vi "SubVI_Protocol_Testing.vi"(0 "TCP Network Connection in":refnum<k5>, 1 "Current level":dbl, 3 "Rest Period":i32=5000, 4 "Max Position":dbl, 5 "error in (no error)":errorcluster, 6 "Target Array":dbl[](array[numeric]), 7 "milliseconds to wait":u32, 9 "MidOut Proportion":dbl=0.6 format="%#_13g", 10 "Arm":string="right", 11 "Fixate Limit":dbl, 12 "Task":i32, 13 "MODE":string, 15 "Move Limit":dbl, 17 "ATAN Limit":dbl=2.0 format="%#_13g", 18 "Imagine Minimum Window":dbl) -> (14 "TCP Network Connection out":refnum<k5>, 19 "error out":errorcluster)   [LabVIEW 2020]
uses:
  Global 1.vi
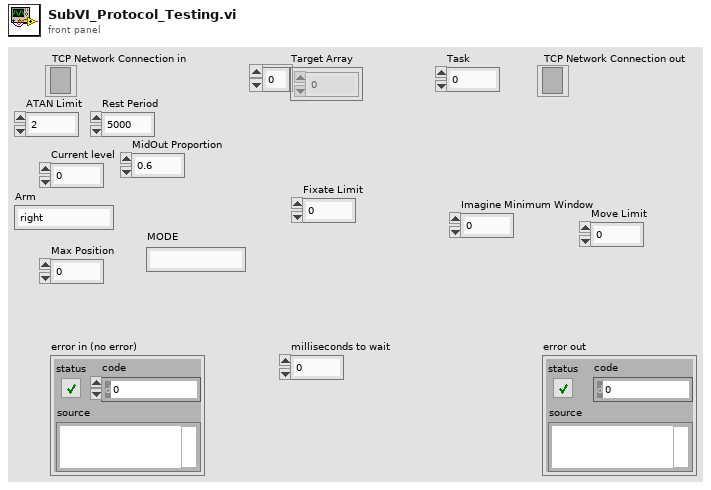
[diagram p1: front panel]
types:
  T1 = enum16{"Standard", "Buffered", "CRLF", "Immediate"}
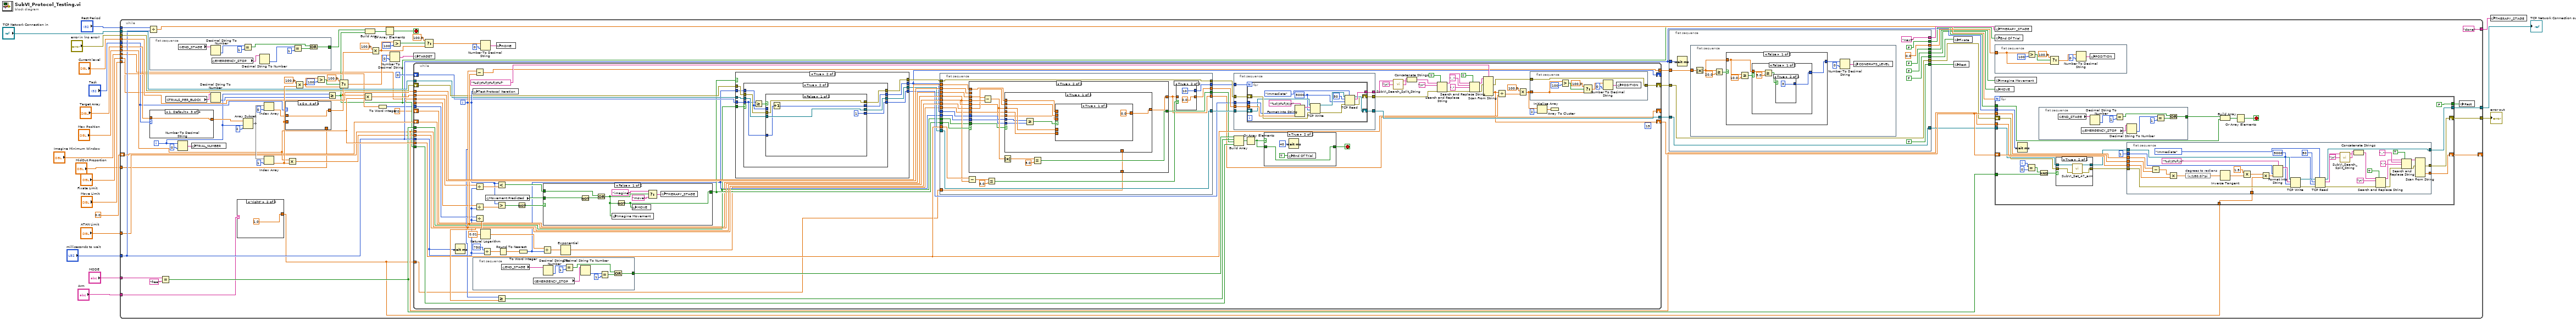
[diagram p0: block diagram]
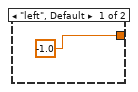
[diagram p2: hidden frame]
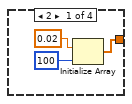
[diagram p3: hidden frame]
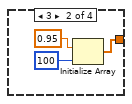
[diagram p4: hidden frame]
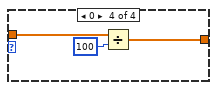
[diagram p5: hidden frame]
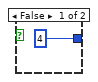
[diagram p6: hidden frame]
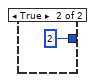
[diagram p7: hidden frame]
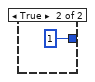
[diagram p8: hidden frame]
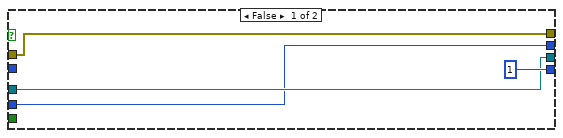
[diagram p10: hidden frame]
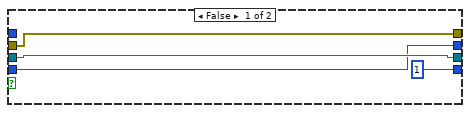
[diagram p11: hidden frame]
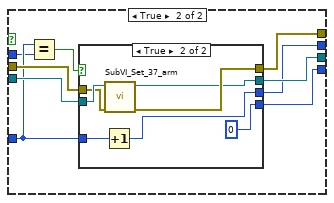
[diagram p12: hidden frame]
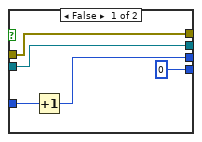
[diagram p13: hidden frame]
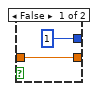
[diagram p15: hidden frame]
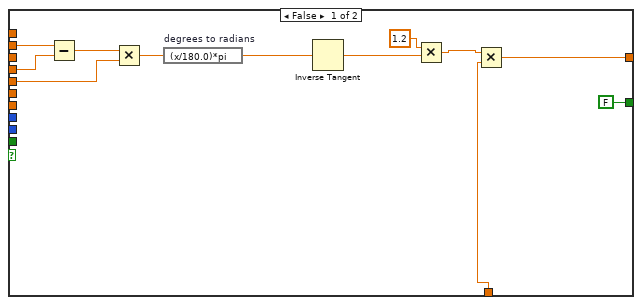
[diagram p16: hidden frame]
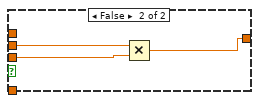
[diagram p17: hidden frame]
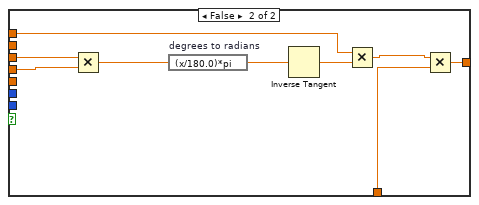
[diagram p18: hidden frame]
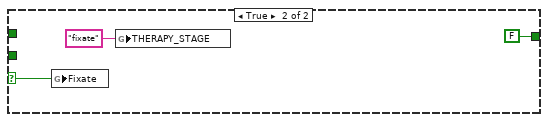
[diagram p19: hidden frame]
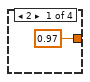
[diagram p20: hidden frame]
diagram:
  n1 = while {
    tunnel: "TCP Network Connection in" -> [w66]
    tunnel: "error in (no error)" -> [w67]
    tunnel: [w61] -> w9
    tunnel: "milliseconds to wait" -> [w53]
    tunnel: "Task" -> [w36]
    tunnel: "Target Array" -> [w38]
    tunnel: ["done" ("THERAPY_STAGE")] -> w10
    tunnel: [w62] -> w11
    tunnel: "Max Position" -> [w64]
    tunnel: "Current level" -> [w63]
    shift-right: [w59] -> _
    shift-left: 0.0 -> [w60]
    tunnel: "ATAN Limit" -> [w30]
    tunnel: "Move Limit" -> [w44]
    tunnel: "Imagine Minimum Window" -> [w27]
    tunnel: "Fixate Limit" -> [w25]
    tunnel: "MODE" -> [w42]
    tunnel: "Rest Period" -> [w28]
    tunnel: "Arm" -> [w22]
    tunnel: "MidOut Proportion" -> [w21]
    i -> [w33]
    stop <- w31 stop-if-true
    n2 = Divide(x=w28, y=w53) -> (x/y=w52:dbl)
    n3 = flat-sequence {
      tunnel: [w471] -> w34
      frame #0 {
        n4 = global read "Global 1.vi" "END_STAGE"() -> (w479:string)
        n5 = Decimal String To Number(string=w479) -> (number=w478:i32)  [unwired: 2 in, 1 out]
        n6 = global read "Global 1.vi" "EMERGENCY_STOP"() -> (w474:string)
        n7 = Equal?(x=w478, y=1) -> (x = y?=w472:bool)
        n8 = Decimal String To Number(string=w474) -> (number=w476:i32)  [unwired: 2 in, 1 out]
        n9 = Equal?(x=w476, y=1) -> (x = y?=w473:bool)
        n10 = Or(x=w472, y=w473) -> (x .or. y?=w471:bool)
      }
    }
    n11 = case shown="1, Default" w36 {
      tunnel: w38 -> [_ _ w104 w107]
      tunnel: [w98 w101 w104 w105] -> w37
      frame 2 {
        n12 = Initialize Array(0.02 ("element"), 100 ("dimension size")) -> (w98:dbl[])
      }
      frame 3 {
        n13 = Initialize Array(0.95 ("element"), 100 ("dimension size")) -> (w101:dbl[])
      }
      frame 1, Default {
      }
      frame 0 {
        n14 = Divide(x=w107, y=100) -> (x/y=w105:dbl[])
      }
    }
    n15 = Equal?(x=w42, y="free") -> (x = y?=w40:bool)
    n16 = global read "Global 1.vi" "TRIALS_PER_BLOCK"() -> (w32:string)
    n17 = Number To Decimal String(number=w33, width (-)=i16 0) -> (decimal integer string=w70:string)
    n18 = global write "Global 1.vi" "TRIAL_NUMBER"(w70) -> ()
    n19 = Decimal String To Number(string=w32) -> (number=w26:i32)  [unwired: 2 in, 1 out]
    n20 = case shown="\"right\"" w22 {
      tunnel: [-1.0 1.0] -> w23
      frame "left", Default {
      }
      frame "right" {
      }
    }
    n21 = Array Subset(array=w37, index=w33, length=2) -> (w94:dbl[])
    n22 = Index Array(array=w94, index=0) -> (element=w73:dbl)
    n23 = Index Array(array=w94, index=1) -> (element=w74:dbl)
    n24 = case shown="0" w36 {
      tunnel: [0.97 0.02 w489 w490] -> w72
      tunnel: w74 -> [_ _ _ _]
      tunnel: w73 -> [_ _ _ w490]
      tunnel: w21 -> [_ _ w489 _]
      frame 2 {
      }
      frame 3 {
      }
      frame 1, Default {
      }
      frame 0 {
      }
    }
    n25 = Multiply(x=w64, y=w74) -> (x*y=w39:dbl)
    n26 = Multiply(x=100.0, y=w74) -> (x*y=w86:dbl)
    n27 = Greater?(x=w86, y=100) -> (0:w90:bool)
    n28 = Greater Or Equal?(x=w33, y=w26) -> (x >= y?=w29:bool)
    n29 = Select(t=100.0, s=w90, f=w86) -> (s? t:f=w91:dbl)
    n30 = Multiply(x=w72, y=w64) -> (x*y=w65:dbl)
    n31 = Build Array(w34, w29) -> (w35:bool[])
    n32 = Multiply(x=100.0, y=w72) -> (x*y=w79:dbl)
    n33 = To Word Integer(number=w44) -> (16bit integer=w20:i16)
    n34 = Or Array Elements(Boolean array=w35) -> (logical OR=w31:bool)
    n35 = Number To Decimal String(number=w91, width (-)=i16 0) -> (decimal integer string=w76:string)
    n36 = Greater?(x=w79, y=100) -> (0:w83:bool)
    n37 = global write "Global 1.vi" "TARGET"(w76) -> ()
    n38 = while {
      tunnel: [w265] -> w54
      shift-right: [w230] -> w56
      shift-left: w67 -> [w243]
      tunnel: w66 -> [w241]
      tunnel: w53 -> [w221]
      tunnel: w65 -> [w258]
      tunnel: w39 -> [w255]
      tunnel: w64 -> [w264]
      shift-right: [w259] -> w58
      shift-left: w60 -> [w254]
      tunnel: w63 -> [w263]
      tunnel: w30 -> [w256]
      tunnel: [w253] -> w46
      tunnel: w20 -> [w247]
      tunnel: w27 -> [w246]
      tunnel: w25 -> [w245]
      tunnel: w40 -> [w228]
      shift-right: [w227] -> _
      shift-left: 0 -> [w238]
      tunnel: w29 -> [w235]
      shift-right: [w226] -> _
      shift-left: 0.0 -> [w225]
      tunnel: w23 -> [w215]
      i -> [w244]
      stop <- w236 stop-if-true
      (unwired) 15 ("y")
      n39 = Wait (ms)(milliseconds to wait=w221) -> ()  [unwired: 1 out]
      n40 = global write "Global 1.vi" "Test Protocol Iteration"(w244) -> ()
      n41 = flat-sequence {
        tunnel: [w443] -> w252
        frame #0 {
          n42 = global read "Global 1.vi" "END_STAGE"() -> (w451:string)
          n43 = global read "Global 1.vi" "EMERGENCY_STOP"() -> (w446:string)
          n44 = Decimal String To Number(string=w451) -> (number=w450:i32)  [unwired: 2 in, 1 out]
          n45 = Equal?(x=w450, y=1) -> (x = y?=w444:bool)
          n46 = Decimal String To Number(string=w446) -> (number=w448:i32)  [unwired: 2 in, 1 out]
          n47 = Equal?(x=w448, y=1) -> (x = y?=w445:bool)
          n48 = Or(x=w444, y=w445) -> (x .or. y?=w443:bool)
        }
      }
      n49 = Subtract(x=w255, y=w254) -> (x-y=w253:dbl)
      n50 = Divide(x=w246, y=w221) -> (x/y=w287:dbl)
      n51 = Divide(x=w245, y=w221) -> (x/y=w288:dbl)
      n52 = Divide(x=w247, y=w221) -> (x/y=w289:dbl)
      n53 = Natural Logarithm(1:0.01 ("y")) -> (0:w223:dbl)
      n54 = Divide(x=750, y=w221) -> (x/y=w218:dbl)
      n55 = global read "Global 1.vi" "Movement Predicted"() -> (w257:bool)
      n56 = Less?(x=w244, y=w287) -> (x < y?=w267:bool)
      n57 = Greater?(x=w244, y=w288) -> (0:w286:bool)
      n58 = Greater Or Equal?(x=w244, y=w289) -> (x >= y?=w251:bool)
      n59 = Round To Nearest(number=w218) -> (nearest integer value=w219:dbl)
      n60 = Not(x=w286) -> (.not. x?=w268:bool)
      n61 = To Word Integer(number=w219) -> (16bit integer=w217:i16)
      n62 = Divide(x=w223, y=w217) -> (x/y=w222:dbl)
      n63 = case shown="False" w268 {
        selector: w268 -> [_ w468]
        tunnel: w257 -> [w466 _]
        tunnel: w267 -> [w465 _]
        tunnel: [w461 FALSE] -> w237
        frame False {
          n64 = Not(x=w466) -> (.not. x?=w460:bool)
          n65 = Or(x=w465, y=w460) -> (x .or. y?=w462:bool)
          n66 = global write "Global 1.vi" "Imagine Movement"(w462) -> ()
          n67 = Not(x=w462) -> (.not. x?=w461:bool)
          n68 = global write "Global 1.vi" "MOVE"(w461) -> ()
          n69 = Select(t="imagine" ("THERAPY_STAGE"), s=w462, f="move" ("THERAPY_STAGE")) -> (s? t:f=w467:string)
          n70 = global write "Global 1.vi" "THERAPY_STAGE"(w467) -> ()
        }
        frame True {
          n71 = global write "Global 1.vi" "Fixate"(w468) -> ()
          n72 = global write "Global 1.vi" "THERAPY_STAGE"("fixate" ("THERAPY_STAGE")) -> ()
        }
      }
      n73 = Exponential(1:w222) -> (0:w216:dbl)
      n74 = case shown="True" w237 {
        tunnel: w243 -> [w292 w302]
        tunnel: [1 ("input 1") w299] -> w242
        tunnel: w241 -> [w291 w296]
        tunnel: [w291 w297] -> w240
        tunnel: [w292 w301] -> w239
        tunnel: w238 -> [w290 w295]
        tunnel: [w290 w300] -> w227
        tunnel: w228 -> [_ w298]
        tunnel: w217 -> [_ w294]
        frame False {
        }
        frame True {
          n75 = case shown="True" w298 {
            tunnel: w302 -> [w306 w315]
            tunnel: w296 -> [w305 w314]
            tunnel: [w305 w313] -> w297
            tunnel: [w306 w312] -> w301
            tunnel: [w303 w311] -> w300
            tunnel: [1 ("input 1") w310] -> w299
            tunnel: w295 -> [w303 w308]
            tunnel: w294 -> [_ w307]
            frame False {
            }
            frame True {
              n76 = Greater Or Equal?(x=w308, y=w307) -> (x >= y?=w309:bool)
              n77 = case shown="False" w309 {
                tunnel: w314 -> [w319 w329]
                tunnel: w315 -> [w320 w328]
                tunnel: [w320 w327] -> w312
                tunnel: [w319 w326] -> w313
                tunnel: [w316 w325] -> w311
                tunnel: [1 ("input 1") w324] -> w310
                tunnel: w308 -> [w317 w323]
                tunnel: w307 -> [_ w322]
                frame False {
                  n78 = Increment(x=w317) -> (x+1=w316:i32)
                }
                frame True {
                  n79 = Equal?(x=w323, y=w322) -> (x = y?=w321:bool)
                  n80 = case shown="True" w321 {
                    tunnel: w329 -> [w332 w341]
                    tunnel: w328 -> [w331 w340]
                    tunnel: [w331 w339] -> w327
                    tunnel: [w332 w338] -> w326
                    tunnel: [w334 w337] -> w325
                    tunnel: [0 ("input 1") 0 ("input 1")] -> w324
                    tunnel: w323 -> [w333 w335]
                    frame False {
                      n81 = Increment(x=w333) -> (x+1=w334:i32)
                    }
                    frame True {
                      n82 = Increment(x=w335) -> (x+1=w337:i32)
                      n83 = call "SubVI_Set_37_arm.vi"("error in (no error)"=w340, "TCP Network Connection in"=w341) -> ("error out"=w339:errorcluster, "TCP Network Connection out"=w338:refnum<k5>)  [unwired: 8 in]
                    }
                  }
                }
              }
            }
          }
        }
      }
      n84 = flat-sequence {
        tunnel: w239 -> [w367]
        tunnel: w240 -> [w366]
        tunnel: w258 -> [w365]
        tunnel: w255 -> [w364]
        tunnel: [w363] -> w261
        tunnel: [w367] -> w260
        tunnel: [w366] -> w262
        tunnel: w254 -> [w354]
        tunnel: w264 -> [w360]
        tunnel: w263 -> [w359]
        tunnel: w237 -> [w358]
        tunnel: w256 -> [w357]
        tunnel: [w356] -> w250
        tunnel: [w355] -> w229
        tunnel: w228 -> [w352]
        tunnel: w227 -> [w351]
        tunnel: w217 -> [w350]
        tunnel: [w349] -> w226
        tunnel: w225 -> [w348]
        tunnel: w216 -> [w347]
        tunnel: w215 -> [w346]
        frame #0 {
          n85 = Subtract(x=w360, y=w354) -> (x-y=w362:dbl)
          n86 = case shown="True" w358 {
            tunnel: w365 -> [w377 _]
            tunnel: w364 -> [_ w395]
            tunnel: w354 -> [w382 w398]
            tunnel: w359 -> [_ w396]
            tunnel: [w378 w397] -> w349
            tunnel: w357 -> [w374 w391]
            tunnel: [FALSE w390] -> w356
            tunnel: w352 -> [_ w389]
            tunnel: w351 -> [_ w388]
            tunnel: w350 -> [_ w387]
            tunnel: w348 -> [_ w386]
            tunnel: w347 -> [_ w385]
            tunnel: w346 -> [w372 w384]
            frame False {
              n87 = Subtract(x=w377, y=w382) -> (x-y=w376:dbl)
              n88 = Multiply(x=w376, y=w374) -> (x*y=w375:dbl)
              n89 = expression code="(x/180.0)*pi" "degrees to radians"(w375) -> (w383:dbl)
              n90 = Inverse Tangent(1:w383) -> (0:w381:dbl)
              n91 = Multiply(x=1.2, y=w381) -> (x*y=w379:dbl)
              n92 = Multiply(x=w379, y=w372) -> (x*y=w378:dbl)
            }
            frame True {
              n93 = Subtract(x=w395, y=w398) -> (x-y=w392:dbl)
              n94 = Absolute Value(x=w392) -> (abs(x)=w394:dbl)
              n95 = case shown="True" w389 {
                tunnel: [w407 w417] -> w397
                tunnel: w396 -> [w406 w416]
                tunnel: w392 -> [w405 w415]
                tunnel: w391 -> [w404 w413]
                tunnel: w388 -> [w403 _]
                tunnel: w387 -> [w402 _]
                tunnel: w386 -> [w400 _]
                tunnel: w385 -> [w399 _]
                tunnel: w384 -> [_ w412]
                frame True {
                  n96 = Greater Or Equal?(x=w403, y=w402) -> (x >= y?=w401:bool)
                  n97 = case shown="True" w401 {
                    tunnel: [0.0 w411] -> w407
                    tunnel: w406 -> [_ _]
                    tunnel: w405 -> [_ _]
                    tunnel: w404 -> [_ _]
                    tunnel: w400 -> [_ w410]
                    tunnel: w399 -> [_ w409]
                    frame True {
                    }
                    frame False {
                      n98 = Multiply(x=w410, y=w409) -> (x*y=w411:dbl)
                    }
                  }
                }
                frame False {
                  n99 = Multiply(x=w415, y=w413) -> (x*y=w414:dbl)
                  n100 = expression code="(x/180.0)*pi" "degrees to radians"(w414) -> (w420:dbl)
                  n101 = Inverse Tangent(1:w420) -> (0:w419:dbl)
                  n102 = Multiply(x=w416, y=w419) -> (x*y=w418:dbl)
                  n103 = Multiply(x=w418, y=w412) -> (x*y=w417:dbl)
                }
              }
              n104 = Less Or Equal?(x=w394, y=5.0) -> (x <= y?=w390:bool)
            }
          }
          n105 = Less Or Equal?(x=w362, y=3.0) -> (x <= y?=w353:bool)
          n106 = case shown="True" w353 {
            tunnel: w349 -> [w369 _]
            tunnel: [w369 0.0] -> w363
            tunnel: [1 10] -> w355
            frame False {
            }
            frame True {
            }
          }
        }
      }
      n107 = flat-sequence {
        tunnel: w261 -> [w428]
        tunnel: [w427] -> w266
        tunnel: [w426] -> w265
        tunnel: [w425] -> w234
        tunnel: w260 -> [w424]
        tunnel: w242 -> [w423]
        tunnel: w262 -> [w422]
        tunnel: w229 -> [w421]
        frame #0 {
          n108 = for {
            N: w421 -> [_]
            tunnel: w428 -> [w436]
            tunnel: [w435] -> w427
            tunnel: w423 -> [w431]
            shift-right: [w433] -> w425
            shift-left: w424 -> [w432]
            shift-right: [w434] -> w426
            shift-left: w422 -> [w430]
            w429 = 5000 ("timeout ms (25000)")
            n109 = Format Into String(format string="%d\\t%f\\t\\n", w431, w436) -> (resulting string=w437:string)  [unwired: 2 in, 1 out]
            n110 = TCP Write(connection ID=w430, data in=w437, error in (no error)=w432, 9:w429) -> (connection ID out=w440:refnum<k5>, error out=w439:errorcluster)  [unwired: 1 out]
            n111 = TCP Read(connection ID=w440, bytes to read=50, error in (no error)=w439, 7:T1."Immediate" ("mode (standard)"), 9:w429) -> (connection ID out=w434:refnum<k5>, data out=w435:string, error out=w433:errorcluster)
          }
        }
      }
      n112 = Build Array(w252, w251, w250, w235) -> (w249:bool[])
      n113 = Or Array Elements(Boolean array=w249) -> (logical OR=w248:bool)
      n114 = case shown="True" w248 {
        tunnel: w248 -> [w342 w345]
        tunnel: [w342 w345] -> w236
        frame False {
        }
        frame True {
          n115 = global write "Global 1.vi" "End Of Trial"(TRUE ("End Of Trial")) -> ()
          n116 = Wait (ms)(milliseconds to wait=u32 40) -> ()  [unwired: 1 out]
        }
      }
      n117 = call <userlib>:"SubVI_Search_Split_String.vi"("search string/char (-)"="\n", "string"=w266) -> ("substring after match"=w280:string, "substring before match"=w271:string)  [unwired: 1 in, 1 out]
      n118 = Concatenate Strings(w280, w271) -> (w277:string)
      n119 = Search and Replace String(replace all?=TRUE ("replace all? (F)"), input string=w277, search string="\n", error in=w234) -> (result string=w272:string, error out=w233:errorcluster)  [unwired: 4 in, 2 out]
      n120 = Search and Replace String(replace all?=TRUE ("replace all? (F)"), input string=w272, search string="..", replace string="." ("replace string (\"\")"), error in=w233) -> (result string=w270:string, error out=w232:errorcluster)  [unwired: 3 in, 2 out]
      n121 = Scan From String(format string="%d\\t%f\\t%f\\t%f", input string=w270, error in=w232) -> (error out=w231:errorcluster, output 3=w259:dbl)  [unwired: 8 in, 2 out]
      n122 = Divide(x=w259, y=w264) -> (x/y=w283:dbl)
      n123 = Multiply(x=100.0, y=w283) -> (x*y=w269:dbl)
      n124 = flat-sequence {
        tunnel: w269 -> [w453]
        tunnel: w231 -> [w452]
        tunnel: [w452] -> w230
        frame #0 {
          n125 = Greater?(x=w453, y=100) -> (0:w458:bool)
          n126 = Select(t=100.0, s=w458, f=w453) -> (s? t:f=w455:dbl)
          n127 = Number To Decimal String(number=w455, width (-)=i16 0) -> (decimal integer string=w454:string)
          n128 = global write "Global 1.vi" "POSITION"(w454) -> ()
        }
      }
      n129 = Initialize Array(w269, 2 ("dimension size")) -> (w284:dbl[])
      n130 = Array To Cluster(array=w284) -> ()  [unwired: 1 out]
    }
    n131 = Select(t=100.0, s=w83, f=w79) -> (s? t:f=w84:dbl)
    n132 = Number To Decimal String(number=w84, width (-)=i16 0) -> (decimal integer string=w77:string)
    n133 = global write "Global 1.vi" "HOME"(w77) -> ()
    n134 = flat-sequence {
      tunnel: [FALSE ("MOVE")] -> w49
      tunnel: [FALSE ("Imagine Movement")] -> w50
      tunnel: [TRUE ("Rest")] -> w47
      tunnel: [FALSE ("Fixate")] -> w51
      tunnel: ["next" ("THERAPY_STAGE")] -> w69
      tunnel: [0.0 ("Arm_position")] -> w68
      tunnel: w53 -> [w112]
      tunnel: [w111] -> w57
      tunnel: w56 -> [w111]
      tunnel: [w110] -> w55
      tunnel: w54 -> [w110]
      tunnel: w46 -> [w109]
      tunnel: [FALSE ("End Of Trial")] -> w45
      frame #0 {
        n135 = Wait (ms)(milliseconds to wait=w112) -> ()  [unwired: 1 out]
        n136 = flat-sequence {
          tunnel: w109 -> [w120]
          frame #0 {
            n137 = Absolute Value(x=w120) -> (abs(x)=w119:dbl)
            n138 = Greater Or Equal?(x=w119, y=20.0) -> (x >= y?=w124:bool)
            n139 = case shown="False" w124 {
              tunnel: [w127 1] -> w122
              tunnel: w119 -> [w126 _]
              frame False {
                n140 = Greater Or Equal?(x=w126, y=10.0) -> (x >= y?=w129:bool)
                n141 = case shown="False" w129 {
                  tunnel: [w131 2] -> w127
                  tunnel: w126 -> [w133 _]
                  frame False {
                    n142 = Greater Or Equal?(x=w133, y=5.0) -> (x >= y?=w130:bool)
                    n143 = case shown="True" w130 {
                      tunnel: [4 3] -> w131
                      frame False {
                      }
                      frame True {
                      }
                    }
                  }
                  frame True {
                  }
                }
              }
              frame True {
              }
            }
            n144 = Number To Decimal String(number=w122, width (-)=i16 0) -> (decimal integer string=w121:string)
            n145 = global write "Global 1.vi" "CONGRATS_LEVEL"(w121) -> ()
          }
        }
      }
    }
    n146 = global write "Global 1.vi" "Fixate"(w51) -> ()
    n147 = global write "Global 1.vi" "Rest"(w47) -> ()
    n148 = global write "Global 1.vi" "THERAPY_STAGE"(w69) -> ()
    n149 = global write "Global 1.vi" "End Of Trial"(w45) -> ()
    n150 = flat-sequence {
      tunnel: w68 -> [w480]
      frame #0 {
        n151 = Greater?(x=w480, y=100) -> (0:w485:bool)
        n152 = Select(t=100.0, s=w485, f=w480) -> (s? t:f=w482:dbl)
        n153 = Number To Decimal String(number=w482, width (-)=i16 0) -> (decimal integer string=w481:string)
        n154 = global write "Global 1.vi" "POSITION"(w481) -> ()
      }
    }
    n155 = global write "Global 1.vi" "Imagine Movement"(w50) -> ()
    n156 = global write "Global 1.vi" "MOVE"(w49) -> ()
    n157 = for {
      N: w52 -> [_]
      shift-right: [w158] -> w61
      shift-left: w57 -> [w146]
      tunnel: [FALSE ("Rest")] -> w48
      tunnel: w55 -> [w145]
      tunnel: [w157] -> w62
      shift-right: [w156] -> w59
      shift-left: w58 -> [w154]
      tunnel: w58 -> [w155]
      tunnel: w53 -> [w153]
      tunnel: w30 -> [w152]
      tunnel: w40 -> [w148]
      tunnel: w29 -> [w140]
      tunnel: w23 -> [w138]
      i -> [w151]
      stop <- w139 stop-if-true
      n158 = Wait (ms)(milliseconds to wait=w153) -> ()  [unwired: 1 out]
      n159 = Equal?(x=w151, y=0) -> (x = y?=w149:bool)
      n160 = flat-sequence {
        tunnel: [w167] -> w141
        frame #0 {
          n161 = global read "Global 1.vi" "END_STAGE"() -> (w175:string)
          n162 = global read "Global 1.vi" "EMERGENCY_STOP"() -> (w170:string)
          n163 = Decimal String To Number(string=w175) -> (number=w174:i32)  [unwired: 2 in, 1 out]
          n164 = Equal?(x=w174, y=1) -> (x = y?=w168:bool)
          n165 = Decimal String To Number(string=w170) -> (number=w172:i32)  [unwired: 2 in, 1 out]
          n166 = Equal?(x=w172, y=1) -> (x = y?=w169:bool)
          n167 = Or(x=w168, y=w169) -> (x .or. y?=w167:bool)
        }
      }
      n168 = And(x=w149, y=w148) -> (x .and. y?=w147:bool)
      n169 = case shown="True" w147 {
        tunnel: w145 -> [w161 w166]
        tunnel: w146 -> [w162 w165]
        tunnel: [w162 w164] -> w143
        tunnel: [w161 w163] -> w144
        frame False {
        }
        frame True {
          n170 = call "SubVI_Set_47_arm.vi"("error in (no error)"=w165, "TCP Network Connection in"=w166) -> ("error out"=w164:errorcluster, "TCP Network Connection out"=w163:refnum<k5>)  [unwired: 8 in]
        }
      }
      n171 = flat-sequence {
        tunnel: 1 ("input 1") -> [w208]
        tunnel: [w207] -> w157
        tunnel: [w178] -> w158
        tunnel: w144 -> [w206]
        tunnel: [w195] -> w156
        tunnel: w155 -> [w192]
        tunnel: w154 -> [w191]
        tunnel: w152 -> [w184]
        tunnel: w143 -> [w182]
        tunnel: w138 -> [w176]
        frame #0 {
          w177 = 5000 ("timeout ms (25000)")
          n172 = Subtract(x=w192, y=w191) -> (x-y=w185:dbl)
          n173 = Multiply(x=w185, y=w184) -> (x*y=w183:dbl)
          n174 = expression code="(x/180.0)*pi" "degrees to radians"(w183) -> (w187:dbl)
          n175 = Inverse Tangent(1:w187) -> (0:w186:dbl)
          n176 = Multiply(x=1.5, y=w186) -> (x*y=w189:dbl)
          n177 = Multiply(x=w189, y=w176) -> (x*y=w190:dbl)
          n178 = Format Into String(format string="%d\\t%f\\n", w208, w190) -> (resulting string=w209:string)  [unwired: 2 in, 1 out]
          n179 = TCP Write(connection ID=w206, data in=w209, error in (no error)=w182, 9:w177) -> (connection ID out=w212:refnum<k5>, error out=w211:errorcluster)  [unwired: 1 out]
          n180 = TCP Read(connection ID=w212, bytes to read=50, error in (no error)=w211, 7:T1."Immediate" ("mode (standard)"), 9:w177) -> (connection ID out=w207:refnum<k5>, data out=w196:string, error out=w181:errorcluster)
          n181 = call <userlib>:"SubVI_Search_Split_String.vi"("search string/char (-)"="\n", "string"=w196) -> ("substring after match"=w204:string, "substring before match"=w198:string)  [unwired: 1 in, 1 out]
          n182 = Concatenate Strings(w204, w198) -> (w202:string)
          n183 = Search and Replace String(replace all?=TRUE ("replace all? (F)"), input string=w202, search string="\n", error in=w181) -> (result string=w199:string, error out=w180:errorcluster)  [unwired: 4 in, 2 out]
          n184 = Search and Replace String(replace all?=TRUE ("replace all? (F)"), input string=w199, search string="..", replace string="." ("replace string (\"\")"), error in=w180) -> (result string=w197:string, error out=w179:errorcluster)  [unwired: 3 in, 2 out]
          n185 = Scan From String(input string=w197, error in=w179) -> (error out=w178:errorcluster, output 3=w195:dbl)  [unwired: 9 in, 2 out]
        }
      }
      n186 = Build Array(w141, w140) -> (w142:bool[])
      n187 = Or Array Elements(Boolean array=w142) -> (logical OR=w139:bool)
    }
    n188 = global write "Global 1.vi" "Rest"(w48) -> ()
  }
  "TCP Network Connection out" <- w11
  "error out" <- w9
  n189 = global write "Global 1.vi" "THERAPY_STAGE"(w10) -> ()
